vi "TL place the boat.vi"(2 "Y pos":i32=100, 3 "X pos":i32=100, 4 "Boat image\nPixels (U32)":u32[][](array[numeric]), 5 "Pool image\nPixels (U32)":u32[][](array[numeric])) -> (0 "Invalid Pos?":bool, 1 "Pool image\nPixels (U32) out":u32[][](array[numeric]))   [LabVIEW 2014]
doc: "This vi will place the boat image in the pool image based upon the X and Y position. It will create a color image array. The position is not valid if the boat is within a solid."
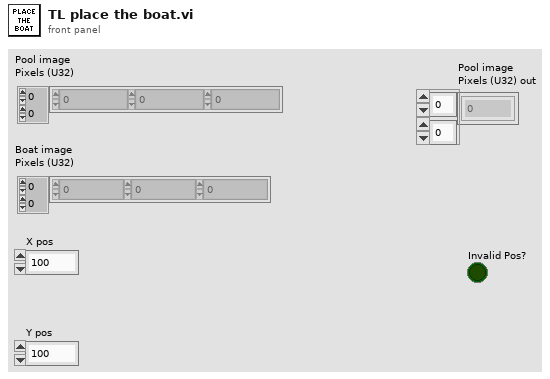
[diagram p1: front panel]
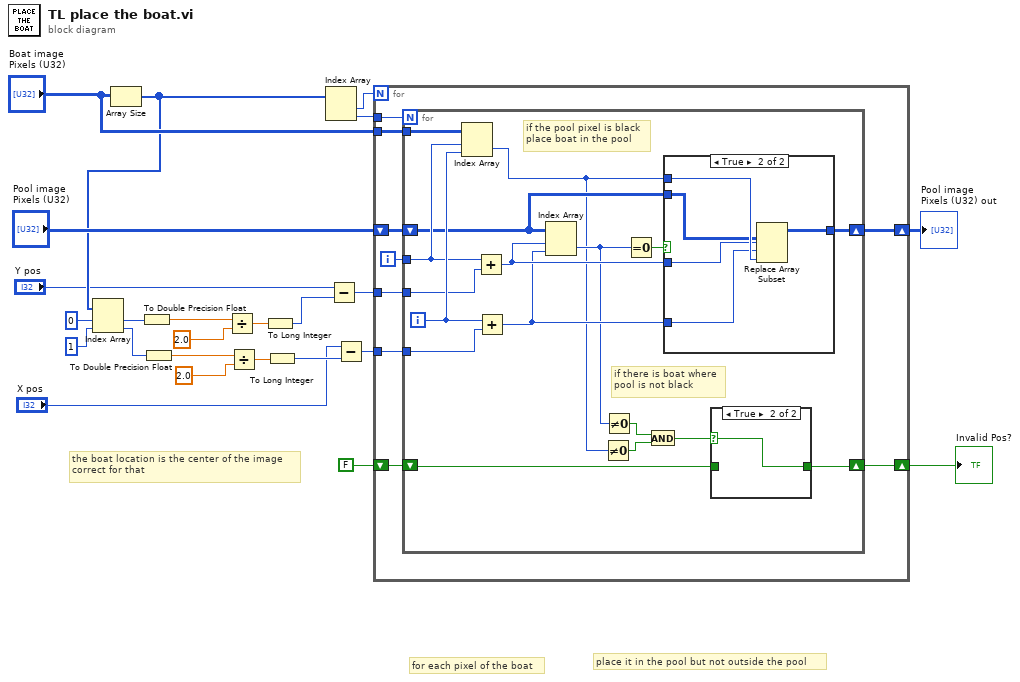
[diagram p0: block diagram]
diagram:
  # "the boat location is the center of the image\ncorrect for that"
  # "place it in the pool but not outside the pool"
  # "for each pixel of the boat"
  n1 = Array Size(array="Boat image\nPixels (U32)") -> (size(s)=w9:i32[])
  n2 = Index Array(array=w9, index #1=0 ("index"), index #2=1 ("index")) -> (element #1=w16:i32, element #2=w12:i32)
  n3 = To Double Precision Float(number=w16) -> (double precision float=w15:dbl)
  n4 = To Double Precision Float(number=w12) -> (double precision float=w13:dbl)
  n5 = Divide(x=w15, y=2.0) -> (x/y=w11:dbl)
  n6 = Divide(x=w13, y=2.0) -> (x/y=w10:dbl)
  n7 = To Long Integer(number=w11) -> (32bit integer=w7:i32)
  n8 = To Long Integer(number=w10) -> (32bit integer=w4:i32)
  n9 = Index Array(array=w9) -> (element #1=w24:i32, element #2=w23:i32)  [unwired: 2 in]
  n10 = Subtract(x="Y pos", y=w7) -> (x-y=w6:i32)
  n11 = Subtract(x="X pos", y=w4) -> (x-y=w5:i32)
  n12 = for {
    N: w24 -> [_]
    tunnel: w23 -> [w32]
    tunnel: "Boat image\nPixels (U32)" -> [w31]
    shift-right: [w29] -> w20
    shift-left: "Pool image\nPixels (U32)" -> [w30]
    tunnel: w6 -> [w28]
    tunnel: w5 -> [w27]
    shift-right: [w25] -> w1
    shift-left: FALSE -> [w26]
    i -> [w33]
    n13 = for {
      N: w32 -> [_]
      tunnel: w33 -> [w48]
      tunnel: w31 -> [w50]
      shift-right: [w47] -> w29
      shift-left: w30 -> [w43]
      tunnel: w28 -> [w42]
      tunnel: w27 -> [w41]
      shift-right: [w34] -> w25
      shift-left: w26 -> [w37]
      i -> [w49]
      # "if there is boat where\npool is not black"
      # "if the pool pixel is black\nplace boat in the pool"
      n14 = Index Array(array=w50, index (row)=w48, index (col)=w49) -> (element=w35:u32)
      n15 = Add(x=w48, y=w42) -> (x+y=w46:i32)
      n16 = Add(x=w49, y=w41) -> (x+y=w45:i32)
      n17 = Index Array(array=w43, index (row)=w46, index (col)=w45) -> (element=w36:u32)
      n18 = Not Equal To 0?(x=w35) -> (x != 0?=w39:bool)
      n19 = Not Equal To 0?(x=w36) -> (x != 0?=w38:bool)
      n20 = Equal To 0?(x=w36) -> (x = 0?=w44:bool)
      n21 = And(x=w38, y=w39) -> (x .and. y?=w40:bool)
      n22 = case shown="True" w44 {
        tunnel: [w53 w58] -> w47
        tunnel: w35 -> [_ w57]
        tunnel: w46 -> [_ w56]
        tunnel: w45 -> [_ w55]
        tunnel: w43 -> [w53 w54]
        frame False {
        }
        frame True {
          n23 = Replace Array Subset(array=w54, new element=w57, index (row)=w56, index (col)=w55) -> (w58:u32[][])
        }
      }
      n24 = case shown="True" w40 {
        selector: w40 -> [_ w52]
        tunnel: w37 -> [w51 _]
        tunnel: [w51 w52] -> w34
        frame False {
        }
        frame True {
        }
      }
    }
  }
  "Pool image\nPixels (U32) out" <- w20
  "Invalid Pos?" <- w1
